vi "Close Ref.vi"(8 "error in (no error)":errorcluster, 11 "Agilent 34401A in":refnum<class "Agilent 34401A.lvclass">) -> (0 "error out":errorcluster, 3 "Agilent 34401A out":refnum<class "Agilent 34401A.lvclass">)   [LabVIEW 2016, in "DMM.lvlib" / "Agilent 34401A.lvclass"]
uses:
  Agilent 34401A.lvclass
  Agilent 34401A.lvclass/Agilent 34401A.ctl
  <instrlib>/Agilent 34401/Agilent 34401.lvlib
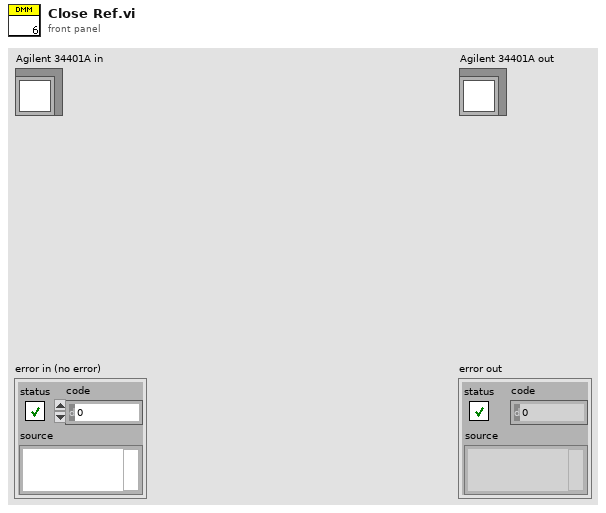
[diagram p1: front panel]
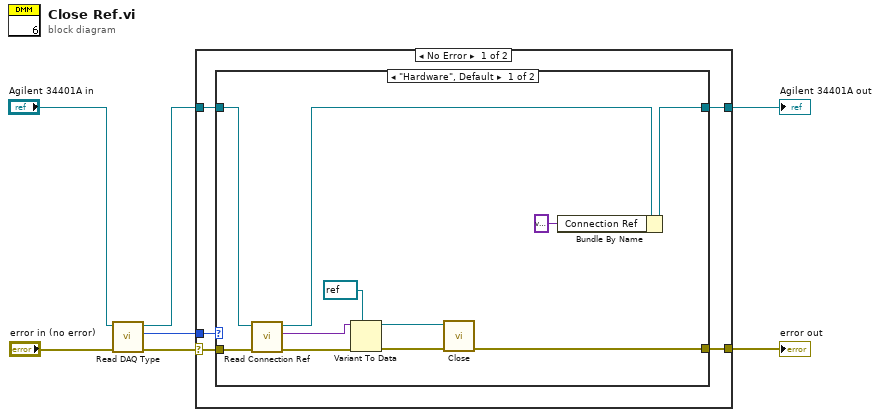
[diagram p0: block diagram]
diagram:
  n1 = call-dynamic "Read DAQ Type.vi"("error in (no error)"="error in (no error)", "Agilent 34401A in"="Agilent 34401A in") -> ("error out"=w6:errorcluster, "DAQ Type"=w5:enum16{"Hardware", "Simulation"}, "Agilent 34401A out"=w1:refnum<class "Agilent 34401A.lvclass">)  [unwired: 7 in]
  n2 = case shown="No Error" w6 {
    selector: w6 -> [w10 w26]
    tunnel: w5 -> [w12 _]
    tunnel: w1 -> [w11 w27]
    tunnel: [w9 w26] -> w3
    tunnel: [w8 w27] -> w2
    frame No Error {
      n3 = case shown="\"Hardware\", Default" w12 {
        tunnel: w11 -> [w15 w25]
        tunnel: w10 -> [w23 w24]
        tunnel: [w17 w24] -> w9
        tunnel: [w16 w25] -> w8
        frame "Hardware", Default {
          n4 = call-dynamic "Read Connection Ref.vi"("error in (no error)"=w23, "Agilent 34401A in"=w15) -> ("error out"=w22:errorcluster, "Connection Ref"=w21:variant, "Agilent 34401A out"=w14:refnum<class "Agilent 34401A.lvclass">)  [unwired: 7 in]
          n5 = Variant To Data(error in=w22, type=refnum<visa-resource-name> refnum ("VISA resource name"), Variant=w21) -> (data=w18:refnum<visa-resource-name>, error out=w20:errorcluster)
          n6 = call <instrlib>:"Close.vi"("error in (no error)"=w20, "VISA resource name"=w18) -> ("error out"=w17:errorcluster)  [unwired: 9 in]
          n7 = Bundle By Name(cluster=w14, "Connection Ref"=variant) -> (w16:refnum<class "Agilent 34401A.lvclass">)
        }
        frame "Simulation" {
        }
      }
    }
    frame Error {
    }
  }
  "error out" <- w3
  "Agilent 34401A out" <- w2
